vi "NIMS_dfd_Convert Band Specs (Remez Constrain).vi"(8 "c":string, 9 "Weight":dbl[](array[numeric]), 10 "A":dbl[](array[numeric]), 11 "F":dbl[](array[numeric])) -> (0 "error out":errorcluster, 2 "band specs":T1[](array[typedef])=[{"band specification"=[{"freq"=0.0, "amplitude"=1.0, "weight"=1.0}, {"freq"=0.2, "amplitude"=1.0, "weight"=1.0}], "ripple constraint"=0.0}, {"band specification"=[{"freq"=0.3, "amplitude"=0.0, "weight"=1.0}, {"freq"=0.5, "amplitude"=0.0, "weight"=1.0}], "ripple constraint"=0.0}])   [LabVIEW 2017, in "NI_DigFilter_MathScript.lvlib"]
uses:
  <vilib>/addons/Digital Filter Design/NI_DigFilter_MathScript.lvlib
  <vilib>/addons/Digital Filter Design/_Objects.llb/DFD Adv Band Spec.ctl
  <vilib>/addons/Digital Filter Design/_Misc.llb/dfd_Error Handlers (Multiple).vi
  <vilib>/addons/Digital Filter Design/NI_DigFilterLicensed.lvlib
panel:
  # "freq"
  # "amplitude"
  # "weight"
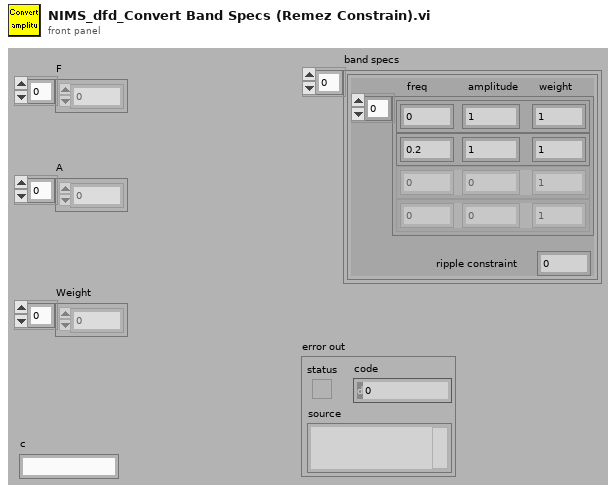
[diagram p1: front panel]
types:
  T1 = typedef "NI_DigFilterLicensed.lvlib/DFD Adv Band Spec.ctl" = cluster{"band specification":cluster{"freq":dbl, "amplitude":dbl, "weight":dbl}[], "ripple constraint":dbl}
  T2 = cluster{"Numeric":dbl, "Numeric":dbl, "Numeric":dbl}
  T3 = cluster{"Numeric":dbl, "Numeric":dbl, "Numeric":dbl}[]
  T4 = cluster{cluster{"Numeric":dbl, "Numeric":dbl, "Numeric":dbl}[], dbl}
  T5 = cluster{cluster{"Numeric":dbl, "Numeric":dbl, dbl}[], "Numeric":dbl}
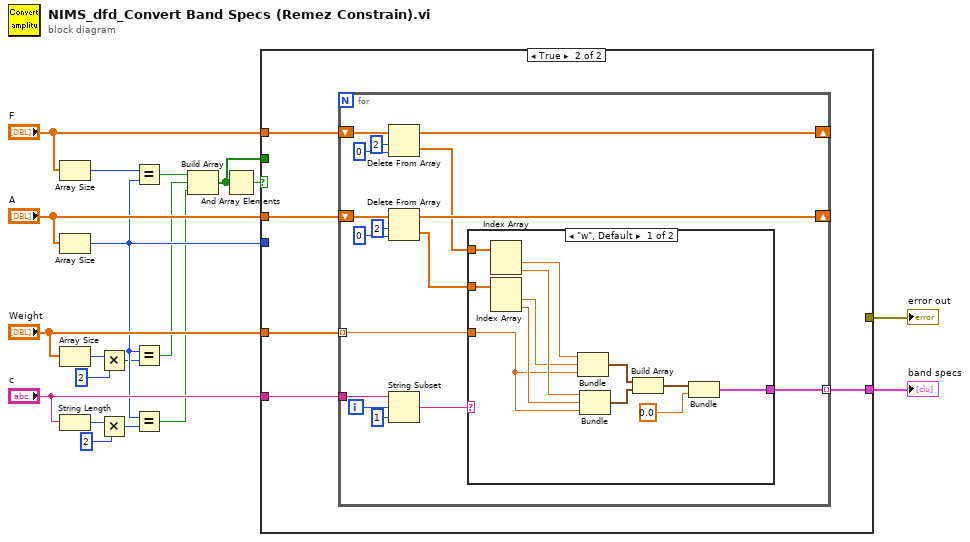
[diagram p0: block diagram]
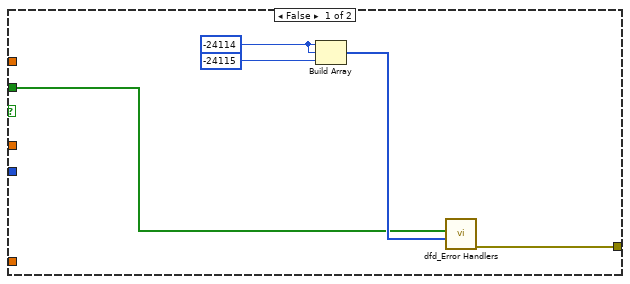
[diagram p2: hidden frame]
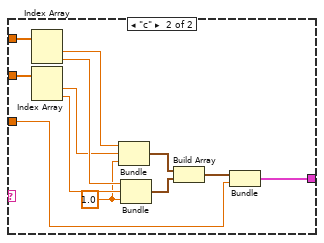
[diagram p3: hidden frame]
diagram:
  n1 = Array Size(array="F") -> (size(s)=w19:i32)
  n2 = Array Size(array="A") -> (size(s)=w13:i32)
  n3 = Array Size(array="Weight") -> (size(s)=w6:i32)
  n4 = String Length(string="c") -> (length=w10:i32)
  n5 = Multiply(x=w6, y=2) -> (x*y=w5:i32)
  n6 = Multiply(x=w10, y=2) -> (x*y=w11:i32)
  n7 = Equal?(x=w19, y=w13) -> (x = y?=w18:bool)
  n8 = Equal?(x=w13, y=w5) -> (x = y?=w7:bool)
  n9 = Equal?(x=w13, y=w11) -> (x = y?=w8:bool)
  n10 = Build Array(w18, w7, w8) -> (w1:bool[])
  n11 = And Array Elements(Boolean array=w1) -> (logical AND=w2:bool)
  n12 = case shown="True" w2 {
    tunnel: "F" -> [_ w29]
    tunnel: "A" -> [_ w28]
    tunnel: "Weight" -> [_ w27]
    tunnel: [w21 _] -> w15
    tunnel: "c" -> [_ w26]
    tunnel: w13 -> [_ _]
    tunnel: [_ w25] -> w3
    tunnel: w1 -> [w20 _]
    frame False {
      w22 = -24114 ("element")
      n13 = Build Array(w22, w22, -24115 ("element")) -> (w24:i32[])
      n14 = call-poly <vilib>:"dfd_Error Handlers.vi"("error sources"=w24, "condition failed?"=w20) -> ("error out"=w21:errorcluster)  [unwired: 1 in, 8 out]
    }
    frame True {
      n15 = for {
        tunnel: w27 -> [w36] mode=indexing
        tunnel: w26 -> [w45]
        shift-right: [w38] -> _
        shift-left: w29 -> [w43]
        shift-right: [w37] -> _
        shift-left: w28 -> [w42]
        tunnel: [w32] -> w25 mode=indexing
        i -> [w41]
        n16 = Delete From Array(array=w43, length=2, index=0) -> (deleted portion=w34:dbl[], array with subset deleted=w38:dbl[])
        n17 = Delete From Array(array=w42, length=2, index=0) -> (deleted portion=w33:dbl[], array with subset deleted=w37:dbl[])
        n18 = String Subset(string=w45, offset (0)=w41, length (rest)=1 ("length (rest)")) -> (substring=w35:string)
        n19 = case shown="\"w\", Default" w35 {
          tunnel: w36 -> [w51 w59]
          tunnel: w33 -> [w56 w68]
          tunnel: w34 -> [w57 w69]
          tunnel: [w46 w60] -> w32
          frame "w", Default {
            n20 = Index Array(array=w57) -> (element #1=w55:dbl, element #2=w54:dbl)  [unwired: 2 in]
            n21 = Index Array(array=w56) -> (element #1=w53:dbl, element #2=w52:dbl)  [unwired: 2 in]
            n22 = Bundle("Numeric"=w55, "Numeric"=w53, "Numeric"=w51) -> (w50:T2)  [unwired: 1 out]
            n23 = Bundle("Numeric"=w54, "Numeric"=w52, "Numeric"=w51) -> (w49:T2)  [unwired: 1 out]
            n24 = Build Array(w50, w49) -> (w48:T3)
            n25 = Bundle(w48, 0.0) -> (w46:T4)  [unwired: 1 out]
          }
          frame "c" {
            w58 = 1.0
            n26 = Index Array(array=w69) -> (element #1=w67:dbl, element #2=w66:dbl)  [unwired: 2 in]
            n27 = Index Array(array=w68) -> (element #1=w65:dbl, element #2=w64:dbl)  [unwired: 2 in]
            n28 = Bundle("Numeric"=w67, "Numeric"=w65, w58) -> (w63:cluster{"Numeric":dbl, "Numeric":dbl, dbl})  [unwired: 1 out]
            n29 = Bundle("Numeric"=w66, "Numeric"=w64, w58) -> (w62:cluster{"Numeric":dbl, "Numeric":dbl, dbl})  [unwired: 1 out]
            n30 = Build Array(w63, w62) -> (w61:cluster{"Numeric":dbl, "Numeric":dbl, dbl}[])
            n31 = Bundle(w61, "Numeric"=w59) -> (w60:T5)  [unwired: 1 out]
          }
        }
      }
    }
  }
  "band specs" <- w3
  "error out" <- w15
